vi "LVFunction_Imop_CameraFile_GetModulePluginName.vi"(0 "HAS file path":path, 11 "error in (no error)":errorcluster) -> (6 "PluginName":string, 15 "error out":errorcluster)   [LabVIEW 2018]
doc: "Get camera interface dll name from configuration file.\n\n--------------------------------------------------------------------------------\n\n<B>config_file_pathIn</B> : Absolute path to Haso or camera configuration file.\n\n<B>config_file_pathOut</B> : Absolute path to Haso or camera configuration file.\n\n<B>plugin_name</B> : Dll name.\n\n<B>ErrorIn</B> : Error\n\n<B>ErrorOut</B> : Error"
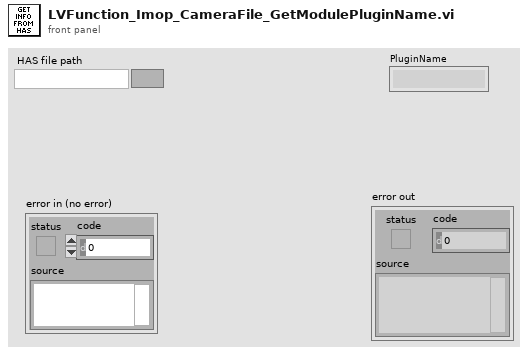
[diagram p1: front panel]
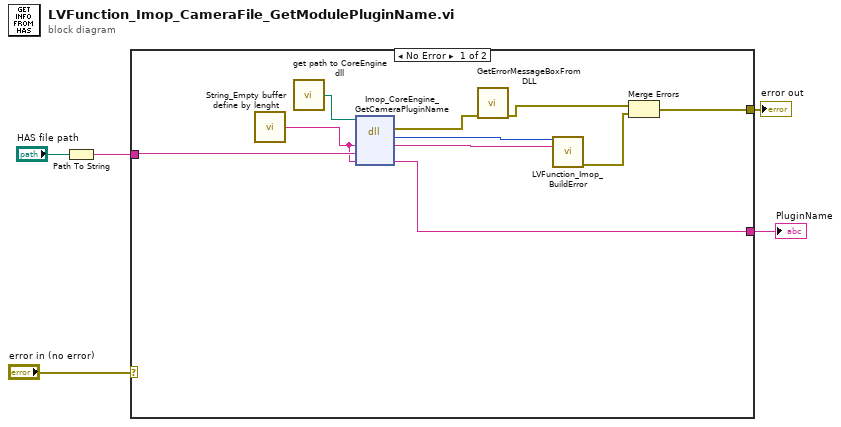
[diagram p0: block diagram]
diagram:
  n1 = Path To String(path="HAS file path") -> (string=w2:string)
  n2 = case shown="No Error" "error in (no error)" {
    selector: "error in (no error)" -> [_ w16]
    tunnel: [w8 w16] -> w4
    tunnel: w2 -> [w11 _]
    tunnel: [w6 _] -> w1
    frame No Error {
      n3 = call "String_Empty buffer define by lenght.vi"() -> ("Empty buffer"=w7:string)  [unwired: 1 in]
      n4 = call "get path to CoreEngine dll.vi"() -> ("path to wavekit library"=w13:path)  [unwired: 14 in, 1 out]
      n5 = dll-call lib="D:/SOFTware/CoreEngine4_Suite/SVN_trunk/LV2011_interface/DLLs/c_interface_vc100.dll" fn="Imop_CoreEngine_GetCameraPluginName"(path in=w13, "message"=w7, "CameraFilePath"=w11, "ModulePluginName"=w7) -> (error out=w12:errorcluster, "return type"=w15:i32, "message"=w14:string, "ModulePluginName"=w6:string)  [unwired: 3 in, 1 out]
      n6 = call "GetErrorMessageBoxFromDLL.vi"("error IN"=w12) -> ("error OUT"=w10:errorcluster)  [unwired: 10 in]
      n7 = call "LVFunction_Imop_BuildError.vi"("code"=w15, "String to Prepend to source (\"\")"=w14) -> ("error out"=w9:errorcluster)  [unwired: 13 in]
      n8 = Merge Errors(w10, w9) -> (w8:errorcluster)
    }
    frame Error {
    }
  }
  "error out" <- w4
  "PluginName" <- w1
